vi "Initialise State.vi"(7 "Part 1?":bool, 8 "error in (no error)":errorcluster, 9 "Sample?":bool, 10 "Sample":string, 11 "Input (use dialog)":path=path "C:/Users/craig.walker/Documents/GitHub/lv2019-Advent-of-Code-2021/23/input.txt") -> (0 "error out":errorcluster, 3 "State out":refnum<class "State.lvclass">)   [LabVIEW 2019, in "23.lvlib" / "State.lvclass"]
uses:
  State.lvclass
  C:/Users/craig.walker/Documents/GitHub/lv2019-LRU-Cache/LRU Node/LRU Node.lvclass
  lv2019-LRU-Cache/LRU Node/LRU Node.lvclass/LRU Node.ctl
  State Key/State Key.lvclass/State Key.ctl
  State Value/State Value.lvclass/State Value.ctl
  lv2019-LRU-Cache/LRU Node/Write Value.vi
  lv2019-LRU-Cache/LRU Node/Read Value.vi
  lv2019-LRU-Cache/LRU Node/Read Key.vi
  lv2019-LRU-Cache/LRU Node/Write Key.vi
  State Key/State Key.lvclass
  State Value/State Value.lvclass
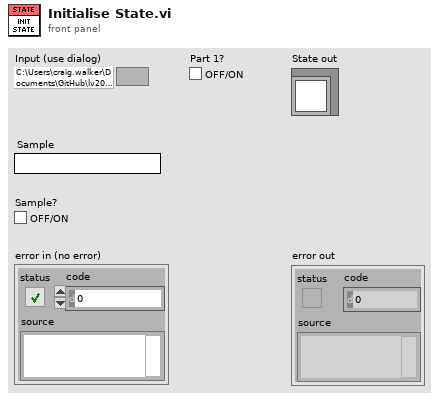
[diagram p1: front panel]
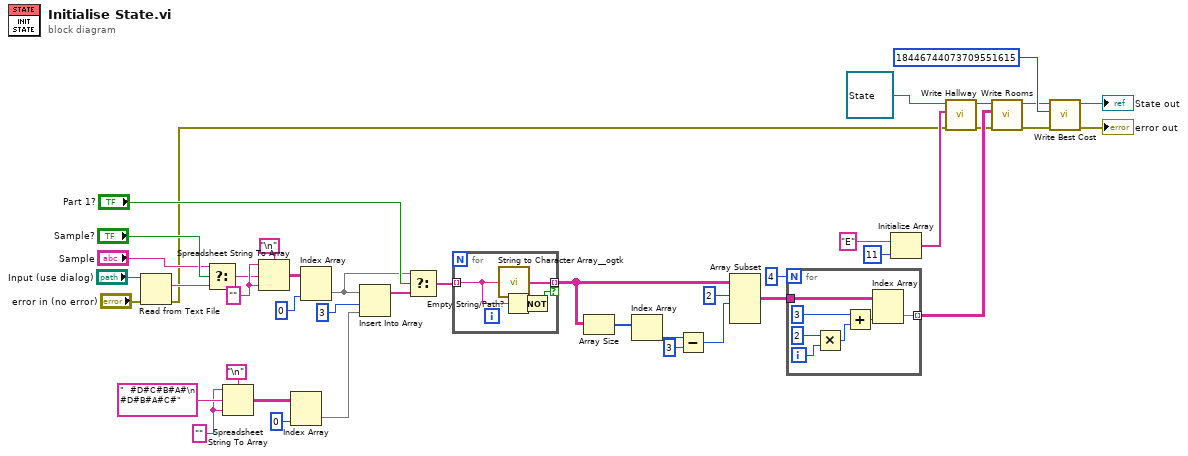
[diagram p0: block diagram]
diagram:
  w23 = "" ("format string")
  w18 = "" ("format string")
  n1 = Read from Text File(file (use dialog)="Input (use dialog)", error in="error in (no error)") -> (text=w14:string, error out=w2:errorcluster)  [unwired: 2 in, 2 out]
  n2 = Select(t="Sample", s="Sample?", f=w14) -> (s? t:f=w17:string)
  n3 = Spreadsheet String To Array(delimiter (Tab)="\n", format string=w23, spreadsheet string="  #D#C#B#A#\n  #D#B#A#C#", array type (2D Dbl)=w23) -> (array=w27:string[][])
  n4 = Spreadsheet String To Array(delimiter (Tab)="\n", format string=w18, spreadsheet string=w17, array type (2D Dbl)=w18) -> (array=w20:string[][])
  n5 = Index Array(array=w27, index (col)=0 ("disabled index (col)")) -> (element=w28:string[])  [unwired: 1 in]
  n6 = Index Array(array=w20, index (col)=0 ("disabled index (col)")) -> (element=w32:string[])  [unwired: 1 in]
  n7 = Insert Into Array(array=w32, index=3, new element=w28) -> (w31:string[])
  n8 = Select(t=w32, s="Part 1?", f=w31) -> (s? t:f=w30:string[])
  n9 = for {
    tunnel: w30 -> [w45] mode=indexing
    tunnel: [w46] -> w34 mode=indexing if=w43
    n10 = call <userlib>:"String to Character Array__ogtk.vi"("Input String"=w45) -> ("Character Array"=w46:string[])
    n11 = Empty String/Path?(string/path=w45) -> (empty?=w44:bool)
    n12 = Not(x=w44) -> (.not. x?=w43:bool)
  }
  n13 = Array Size(array=w34) -> (size(s)=w35:i32[])
  n14 = Index Array(array=w35) -> (element=w38:i32)  [unwired: 1 in]
  n15 = Subtract(x=w38, y=3) -> (x-y=w39:i32)
  n16 = Array Subset(array=w34, index (row)=2, length (row)=w39) -> (w37:string[][])  [unwired: 2 in]
  n17 = for {
    N: 4 -> [_]
    tunnel: w37 -> [w53]
    tunnel: [w47] -> w10 mode=indexing
    i -> [w50]
    n18 = Multiply(x=2, y=w50) -> (x*y=w48:i32)
    n19 = Add(x=3 ("disabled index (col)"), y=w48) -> (x+y=w51:i32)
    n20 = Index Array(array=w53, index (col)=w51) -> (element=w47:string[])  [unwired: 1 in]
  }
  n21 = Initialize Array("E", 11 ("dimension size")) -> (w6:string[])
  n22 = call "Write Hallway.vi"("error in (no error)"=w2, "Hallway"=w6, "State in"=refnum<class "State.lvclass"> refnum ("23.lvlib:State.lvclass")) -> ("error out"=w5:errorcluster, "State out"=w8:refnum<class "State.lvclass">)  [unwired: 7 in]
  n23 = call "Write Rooms.vi"("error in (no error)"=w5, "Rooms"=w10, "State in"=w8) -> ("error out"=w4:errorcluster, "State out"=w7:refnum<class "State.lvclass">)  [unwired: 7 in]
  n24 = call "Write Best Cost.vi"("error in (no error)"=w4, "Best Cost"=u64 18446744073709551615, "State in"=w7) -> ("error out"=→"error out":errorcluster, "State out"=→"State out":refnum<class "State.lvclass">)  [unwired: 7 in]
